vi "Init.vi"(11 "WebView2 Updater in":refnum<class "WebView2 Updater.lvclass">) -> (0 "error out":errorcluster, 3 "WebView2 Updater out":refnum<class "WebView2 Updater.lvclass">)   [LabVIEW 2020, in "WebView2 Updater.lvclass"]
uses:
  WebView2 Updater.lvclass
  WebView2 Updater.lvclass/WebView2 Updater.ctl
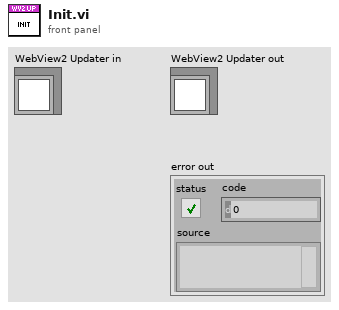
[diagram p1: front panel]
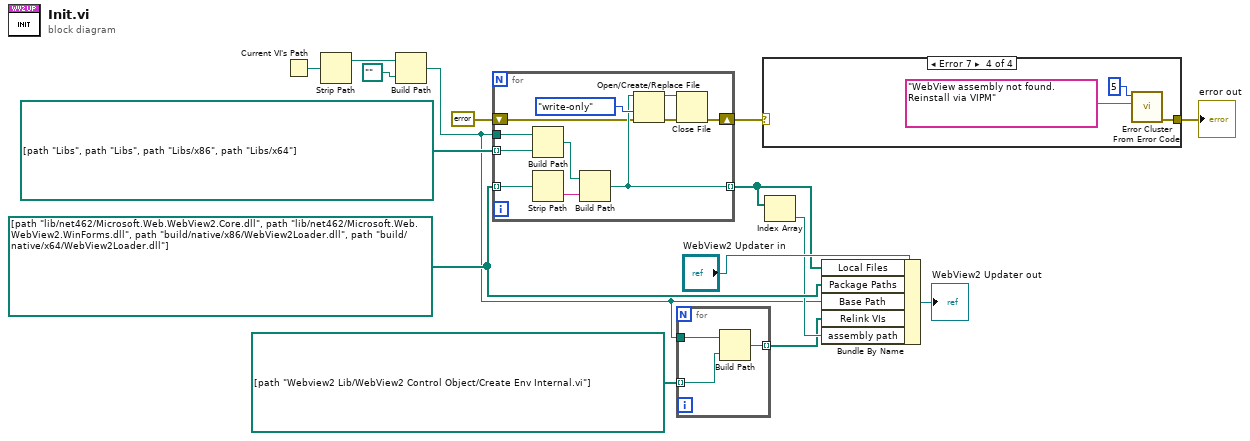
[diagram p0: block diagram]
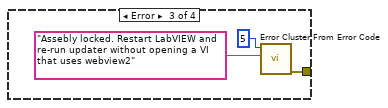
[diagram p4: hidden frame]
diagram:
  w10 = path[] [path "lib/net462/Microsoft.Web.WebView2.Core.dll", path "lib/net462/Microsoft.Web.WebView2.WinForms.dll", path "build/native/x86/WebView2Loader.dll", path "build/native/x64/WebView2Loader.dll"] ("Package Paths")
  n1 = Current VI's Path() -> (path=w11:path)
  n2 = Strip Path(path=w11) -> (stripped path=w5:path)  [unwired: 1 out]
  n3 = Build Path(base path=w5, name or relative path=path "..") -> (appended path=w3:path)
  n4 = for {
    tunnel: [w20] -> w7 mode=indexing
    tunnel: path[] [path "Libs", path "Libs", path "Libs/x86", path "Libs/x64"] ("Local Files") -> [w22] mode=indexing
    tunnel: w10 -> [w21] mode=indexing
    tunnel: w3 -> [w17]
    shift-right: [w18] -> w9
    shift-left: errorcluster {"status"=FALSE, "code"=0, "source"=""} ("error out") -> [w16]
    n5 = Build Path(base path=w17, name or relative path=w22) -> (appended path=w23:path)
    n6 = Strip Path(path=w21) -> (name=w19:string)  [unwired: 1 out]
    n7 = Build Path(base path=w23, name or relative path=w19) -> (appended path=w20:path)
    n8 = Open/Create/Replace File(file path (use dialog)=w20, error in=w16, access (0:read/write)=enum16{"read/write", "read-only", "write-only"}."write-only") -> (refnum out=w26:refnum<file>, error out=w25:errorcluster)  [unwired: 3 in, 1 out]
    n9 = Close File(refnum=w26, error in=w25) -> (error out=w18:errorcluster)  [unwired: 1 out]
  }
  n10 = for {
    tunnel: w3 -> [w29]
    tunnel: path[] [path "Webview2 Lib/WebView2 Control Object/Create Env Internal.vi"] ("Local Files") -> [w28] mode=indexing
    tunnel: [w27] -> w1 mode=indexing
    n11 = Build Path(base path=w29, name or relative path=w28) -> (appended path=w27:path)
  }
  n12 = case shown="Error 7" w9 {
    selector: w9 -> [_ w30 _ _]
    tunnel: [_ w30 w31 w34] -> w14
    frame No Error {
    }
    frame Default {
    }
    frame Error {
      n13 = call <vilib>:"Error Cluster From Error Code.vi"("error message (\"\")"="Assebly locked. Restart LabVIEW and re-run updater without opening a VI that uses webview2" ("error message (\"\")"), "error code (0)"=5) -> ("error out"=w31:errorcluster)  [unwired: 7 in]
    }
    frame Error {
      n14 = call <vilib>:"Error Cluster From Error Code.vi"("error message (\"\")"="WebView assembly not found. Reinstall via VIPM" ("error message (\"\")"), "error code (0)"=5) -> ("error out"=w34:errorcluster)  [unwired: 7 in]
    }
  }
  "error out" <- w14
  n15 = Index Array(array=w7) -> (element=w6:path)  [unwired: 1 in]
  n16 = Bundle By Name(cluster="WebView2 Updater in", "Local Files"=w7, "Package Paths"=w10, "Base Path"=w3, "Relink VIs"=w1, "assembly path"=w6) -> (→"WebView2 Updater out":refnum<class "WebView2 Updater.lvclass">)
